vi "DHE_ResetobsID.vi"(8 "error in (no error)":errorcluster) -> (0 "error out":errorcluster)   [LabVIEW 2016]
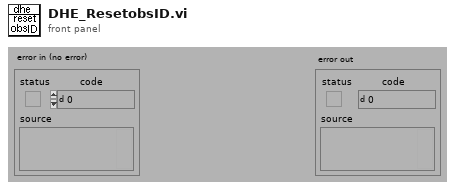
[diagram p1: front panel]
types:
  T1 = typedef "DatabaseHand_RefNum.ctl" = refnum<vi>
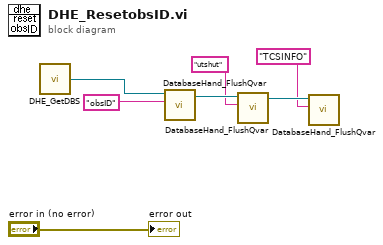
[diagram p0: block diagram]
diagram:
  n1 = call "DHE_GetDBS.vi"() -> ("DHE_DBSRef"=w5:T1)  [unwired: 9 out]
  n2 = call "DatabaseHand_FlushQvar.vi"("name"="obsID", "Database RefNum In"=w5) -> ("Database RefNum out"=w4:T1)  [unwired: 1 in, 8 out]
  n3 = call "DatabaseHand_FlushQvar.vi"("name"="utshut", "Database RefNum In"=w4) -> ("Database RefNum out"=w2:T1)  [unwired: 1 in, 8 out]
  n4 = call "DatabaseHand_FlushQvar.vi"("name"="TCSINFO", "Database RefNum In"=w2) -> ()  [unwired: 1 in, 9 out]
  "error out" <- "error in (no error)"
